vi "Insert Conditional Branch.vi"(6 "Insertion Index":i32=-1, 7 "Parent ID":string, 8 "error in (no error)":errorcluster, 9 "Unique ID":string, 10 "Name":string, 11 "Custom Type Test Executive in":refnum<class "Custom Type Test Executive.lvclass">) -> (0 "error out":errorcluster, 1 "Replaced?":bool, 3 "Custom Type Test Executive out":refnum<class "Custom Type Test Executive.lvclass">, 5 "Unique ID out":string)   [LabVIEW 2017, in "Custom Type Test Executive.lvlib" / "Custom Type Test Executive.lvclass"]
uses:
  <vilib>/gpm_packages/@cs/test-executive/Source/Custom Type Test Executive/Custom Type Test Executive/Custom Type Test Executive.lvclass
  C:/Program Files/National Instruments/LabVIEW 2017/vi.lib/gpm_packages/@cs/test-executive/Source/Test Executive/TestExecutive/Test Executive.lvclass
  <vilib>/gpm_packages/@cs/test-executive/Source/Test Executive/Conditional Branch/Conditional Branch.lvclass
  <vilib>/gpm_packages/@cs/data-type-serializer/source/Boolean/Boolean.lvclass/Boolean.ctl
  <vilib>/gpm_packages/@cs/test-executive/Source/Test Executive/TestExecutive/Test Executive.lvclass/Test Executive.ctl
  cc607d6a-6b14-43bc-b699-5576d5b9cf29.vi
  <vilib>/gpm_packages/@cs/data-type-serializer/source/Boolean/Boolean.lvclass
  <vilib>/gpm_packages/@cs/linked-list/Source/Linked List/ILinkedList/ILinked List.lvclass
  <vilib>/gpm_packages/@cs/linked-list/Source/Linked List/Linked List Ref/Linked List Ref.lvclass
  <vilib>/gpm_packages/@cs/test-executive/Source/Test Executive/TestExecutive/Test Executive.lvclass
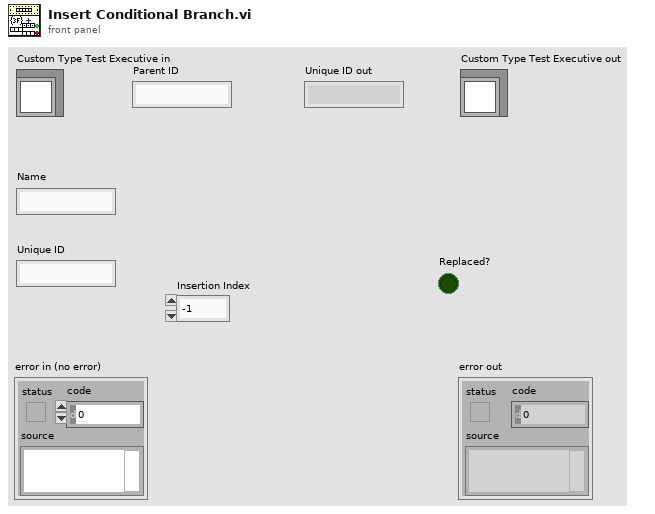
[diagram p1: front panel]
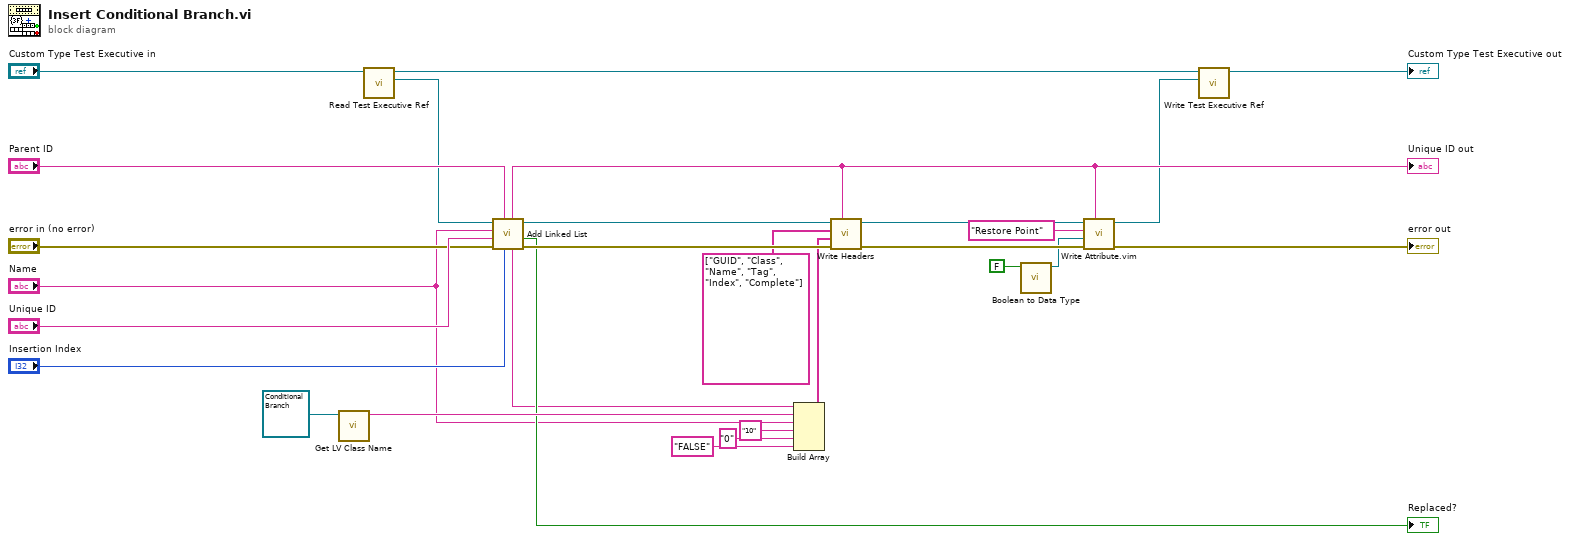
[diagram p0: block diagram]
diagram:
  n1 = call <vilib>:"Get LV Class Name.vi"("object"=refnum<class "Conditional Branch.lvclass"> refnum ("Test Executive.lvlib:Conditional Branch.lvclass")) -> ("class name"=w24:string)  [unwired: 9 in, 1 out]
  n2 = call <vilib>:"Read Test Executive Ref.vi"("Test Executive in"="Custom Type Test Executive in") -> ("Test Executive Ref"=w6:refnum<data-value>, "Test Executive out"=w5:refnum<class "Custom Type Test Executive.lvclass">)  [unwired: 9 in]
  n3 = call <vilib>:"Add Linked List.vi"("Insertion Index"="Insertion Index", "Parent ID"="Parent ID", "error in (no error)"="error in (no error)", "Linked List ID"="Unique ID", "Name"="Name", "Linked List Ref"=w6) -> ("error out"=w26:errorcluster, "Replaced?"=→"Replaced?":bool, "Linked List Ref out"=w27:refnum<data-value>, "Linked List ID out"=w13:string)  [unwired: 2 in]
  "Unique ID out" <- w13
  n4 = Build Array(w13, w24, "Name", "10" ("element"), "0" ("element"), "FALSE" ("element")) -> (w22:string[])
  n5 = call <vilib>:"Write Headers.vi"("Linked List ID"=w13, "error in (no error)"=w26, "Header Values"=w22, "Header Names"=string[] ["GUID", "Class", "Name", "Tag", "Index", "Complete"], "Linked List Ref"=w27) -> ("error out"=w19:errorcluster, "Linked List Ref out"=w20:refnum<data-value>)  [unwired: 5 in]
  n6 = call <vilib>:"Boolean to Data Type.vi"("Boolean"=FALSE) -> ("Boolean out"=w1:refnum<class "Boolean.lvclass">)  [unwired: 9 in, 1 out]
  n7 = call "Write Attribute.vim"("Linked List ID"=w13, "error in (no error)"=w19, "Attribute"=w1, "Attribute Name"="Restore Point", "Linked List Ref"=w20) -> ("error out"=→"error out":errorcluster, "Linked List Ref out"=w3:refnum<data-value>)  [unwired: 3 in, 2 out]
  n8 = call <vilib>:"Write Test Executive Ref.vi"("Test Executive Ref"=w3, "Test Executive in"=w5) -> ("Test Executive out"=→"Custom Type Test Executive out":refnum<class "Custom Type Test Executive.lvclass">)  [unwired: 9 in]
